vi "PiezoDriverWDAQ.vi"() -> ()   [LabVIEW 2017]
panel:
  in  "Set Voltage to 1":bool
  in  "Increase Voltage":bool=TRUE
  in  "Set Voltage to 0":bool
  in  "?":bool
  out "Intesity VS Voltage":cluster{dbl[], dbl[]}[](graph)
  out "Voltage Out VS Voltage In":cluster{dbl[], dbl[]}(graph)
  out "Error Out":errorcluster
  in  "Data Collection\nTime  Interval (ms)":u32=1
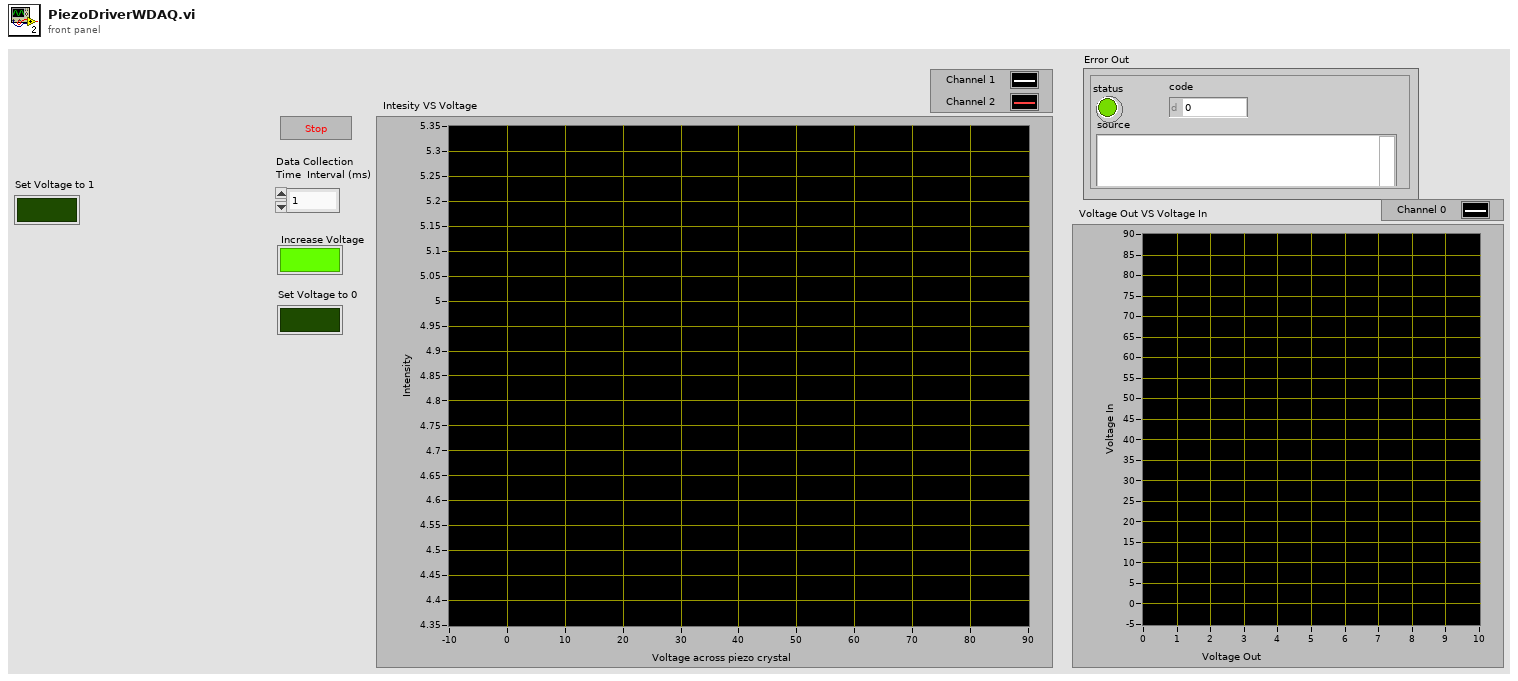
[diagram p1: front panel]
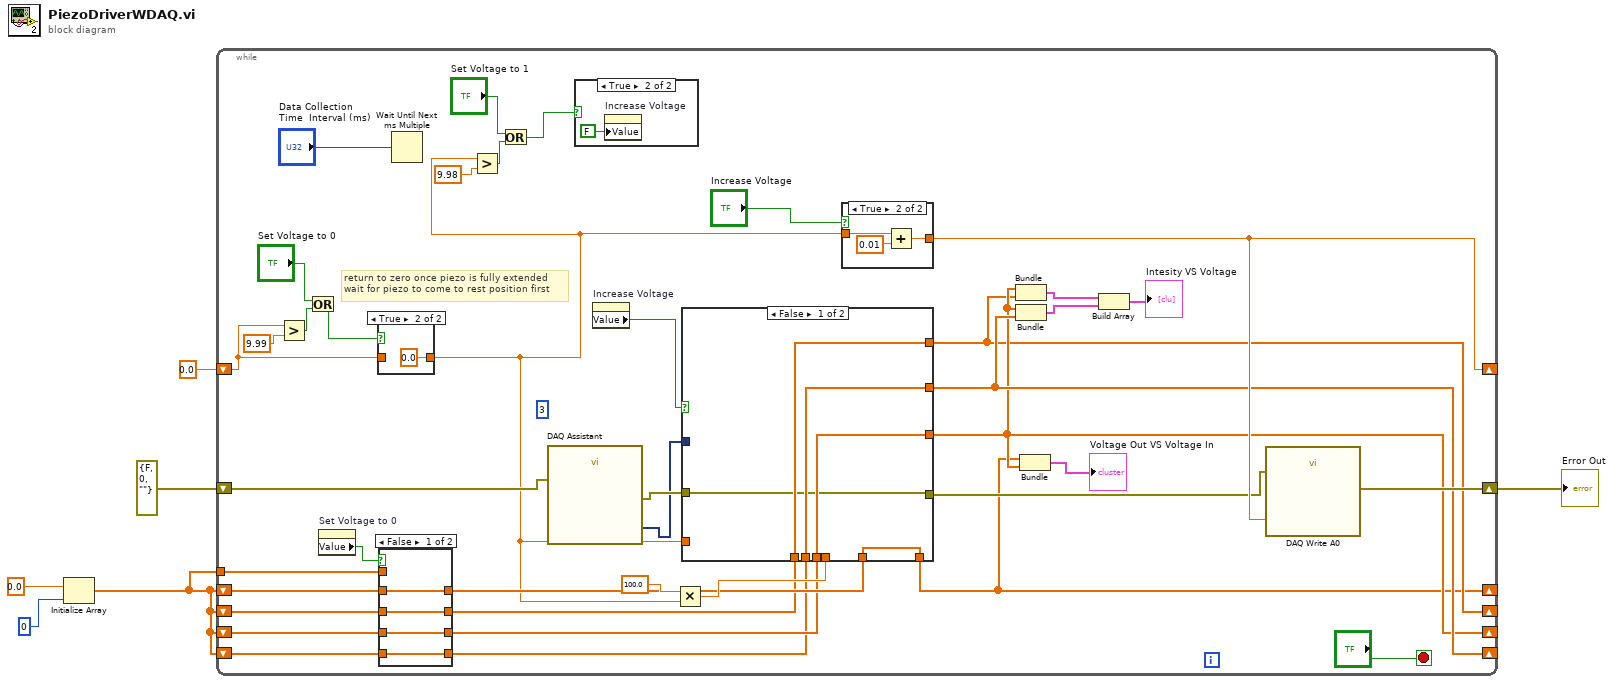
[diagram p0: block diagram]
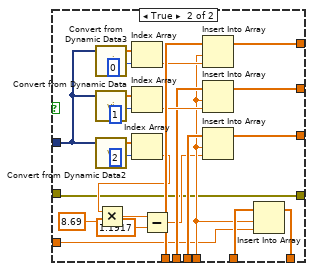
[diagram p4: hidden frame]
diagram:
  n1 = Initialize Array(0.0 ("element"), 0 ("dimension size")) -> (w2:dbl[])
  n2 = while {
    shift-right: [w35] -> w1
    shift-left: errorcluster {"status"=FALSE, "code"=0, "source"=""} ("Error In") -> [w14]
    shift-right: [w16] -> _
    shift-left: w2 -> [w17]
    shift-right: [w15] -> _
    shift-left: w2 -> [w18]
    shift-right: [w20] -> _
    shift-left: w2 -> [w21]
    shift-right: [w27] -> _
    shift-left: w2 -> [w31]
    shift-right: [w36] -> _
    shift-left: 0.0 -> [w44]
    tunnel: w2 -> [w29]
    stop <- "?" stop-if-true
    (unwired) 3 ("number of samples")
    # "return to zero once piezo is fully extended\nwait for piezo to come to rest position first"
    n3 = Greater?(x=w44, y=9.99) -> (0:w43:bool)
    n4 = Or(x="Set Voltage to 0", y=w43) -> (x .or. y?=w42:bool)
    n5 = property on="Set Voltage to 0" class="Bool (strict)"() -> ("Value"=w22:bool)  [unwired: 2 in, 2 out]
    n6 = case shown="True" w42 {
      tunnel: [w87 0.0] -> w9
      tunnel: w44 -> [w87 _]
      frame False {
      }
      frame True {
      }
    }
    n7 = case shown="False" w22 {
      tunnel: [w51 w52] -> w34
      tunnel: w18 -> [w51 _]
      tunnel: w17 -> [w50 _]
      tunnel: [w50 w52] -> w33
      tunnel: w21 -> [w48 _]
      tunnel: [w48 w52] -> w32
      tunnel: [w49 w52] -> w30
      tunnel: w31 -> [w49 _]
      tunnel: w29 -> [_ w52]
      frame False {
      }
      frame True {
      }
    }
    n8 = Wait Until Next ms Multiple(millisecond multiple="Data Collection\nTime  Interval (ms)") -> ()  [unwired: 1 out]
    n9 = Greater?(x=w9, y=9.98) -> (0:w11:bool)
    n10 = Or(x="Set Voltage to 1", y=w11) -> (x .or. y?=w7:bool)
    n11 = call "DAQ Assistant"("error in"=w14) -> ("data"=w12:dynamicdata, "error out"=w13:errorcluster)  [unwired: 16 in, 1 out]
    n12 = case shown="True" w7 {
      frame False {
      }
      frame True {
        n13 = property on="Increase Voltage" class="Bool (strict)"("Value"=FALSE ("Increase Voltage")) -> ()  [unwired: 2 in, 2 out]
      }
    }
    n14 = property on="Increase Voltage" class="Bool (strict)"() -> ("Value"=w37:bool)  [unwired: 2 in, 2 out]
    n15 = Multiply(x=100.0 ("y"), y=w9) -> (x*y=w38:dbl)
    n16 = case shown="False" w37 {
      tunnel: w32 -> [w55 w82]
      tunnel: [w55 w60] -> w20
      tunnel: w33 -> [w57 w81]
      tunnel: [w56 w78] -> w27
      tunnel: [w57 w77] -> w16
      tunnel: w30 -> [w56 w73]
      tunnel: w12 -> [_ w72]
      tunnel: w38 -> [_ w63]
      tunnel: w34 -> [w54 w64]
      tunnel: w9 -> [_ w62]
      tunnel: [w54 w61] -> w15
      tunnel: w13 -> [w53 w58]
      tunnel: [w53 w58] -> w19
      frame False {
      }
      frame True {
        n17 = call "Convert from Dynamic Data3"("Dynamic Data Type"=w72) -> ("Array"=w69:dbl[])  [unwired: 3 in]
        n18 = call "Convert from Dynamic Data"("Dynamic Data Type"=w72) -> ("Array"=w71:dbl[])  [unwired: 3 in]
        n19 = call "Convert from Dynamic Data2"("Dynamic Data Type"=w72) -> ("Array"=w70:dbl[])  [unwired: 3 in]
        n20 = Index Array(array=w69, index=0) -> (element=w80:dbl)
        n21 = Index Array(array=w71, index=1) -> (element=w79:dbl)
        n22 = Index Array(array=w70, index=2) -> (element=w65:dbl)
        n23 = Multiply(x=w65, y=8.69) -> (x*y=w68:dbl)
        n24 = Subtract(x=w68, y=1.1917) -> (x-y=w59:dbl)
        n25 = Insert Into Array(array=w81, index=w63, new element=w80) -> (w77:dbl[])
        n26 = Insert Into Array(array=w73, index=w63, new element=w79) -> (w78:dbl[])
        n27 = Insert Into Array(array=w82, index=w63, new element=w59) -> (w60:dbl[])
        n28 = Insert Into Array(array=w64, index=w63, new element=w62) -> (w61:dbl[])
      }
    }
    n29 = case shown="True" "Increase Voltage" {
      tunnel: [w83 w86] -> w36
      tunnel: w9 -> [w83 w85]
      frame False {
      }
      frame True {
        n30 = Add(x=w85, y=0.01) -> (x+y=w86:dbl)
      }
    }
    n31 = Bundle(w20, w16) -> (w25:cluster{dbl[], dbl[]})  [unwired: 1 in]
    n32 = Bundle(w20, w27) -> (w26:cluster{dbl[], dbl[]})  [unwired: 1 in]
    n33 = Bundle(w15, w20) -> (→"Voltage Out VS Voltage In":cluster{dbl[], dbl[]})  [unwired: 1 in]
    n34 = Build Array(w25, w26) -> (→"Intesity VS Voltage":cluster{dbl[], dbl[]}[])
    n35 = call "DAQ Write A0"("data"=w36, "error in"=w19) -> ("error out"=w35:errorcluster)  [unwired: 16 in, 1 out]
  }
  "Error Out" <- w1
